vi "Read Dashboard Variables.vi"() -> ()   [LabVIEW 2020]
uses:
  <vilib>/Rock Robotics/Network Tables/NT Read Number.vi
  Framework/Robot Global Data.vi
  <vilib>/Rock Robotics/Network Tables/NT Read String.vi
panel:
  out "MaxDrive":dbl(slide)=0.6824817518248175 min=0.0 max=1.0 step=0.01 scale=0.0..1.0
  out "DriveK":dbl(slide)=0.26277372262773724 min=0.0 max=1.0 step=0.05 scale=0.0..1.0
  out "Limelight Goal Area":dbl(slide)=14.8723 min=0.1 max=25.0 step=0.25 scale=0.0..25.0
  out "AimDeadband":dbl min=0.0 max=10.0 step=0.25
  out "MinSteerCommand":dbl(slide)=0.2717391304347826 min=0.0 max=0.5 step=0.05 scale=0.0..0.5
  out "SteeringK":dbl(slide)=0.025362318840579712 min=0.0 max=0.25 step=0.01 scale=0.0..0.25
  out "Shooter Setpoint Reverse":dbl=0.8 format="%#_13g"
  out "Transfer Release Setpoint Reverse":dbl
  out "Intake Reverse Setpoint":dbl=0.8 format="%#_13g"
  out "Reverse Duration":dbl=3.0 format="%#_13g"
  out "Intake Sped Up Setpoint":dbl=0.8 format="%#_13g"
  out "Intake Sped Up Duration":dbl=3.0 format="%#_13g"
  out "Custom MaxSpeedSlow (0.6)":dbl=0.6
  out "Transfer Release Duration":dbl
  out "Transfer Up Duration":dbl
  out "Pivot Duration":dbl
  out "Pivot Right Speed":dbl
  out "Pivot Left Speed":dbl
  out "Transfer Release Setpoint":dbl
  out "Transfer Up Setpoint":dbl
  out "Intake Setpoint":dbl=0.8 format="%#_13g"
  out "Intake Duration (s)":dbl=3.0 format="%#_13g"
  out "Shooter Duration":dbl=3.0 format="%#_13g"
  out "Shooter Setpoint":dbl=0.8 format="%#_13g"
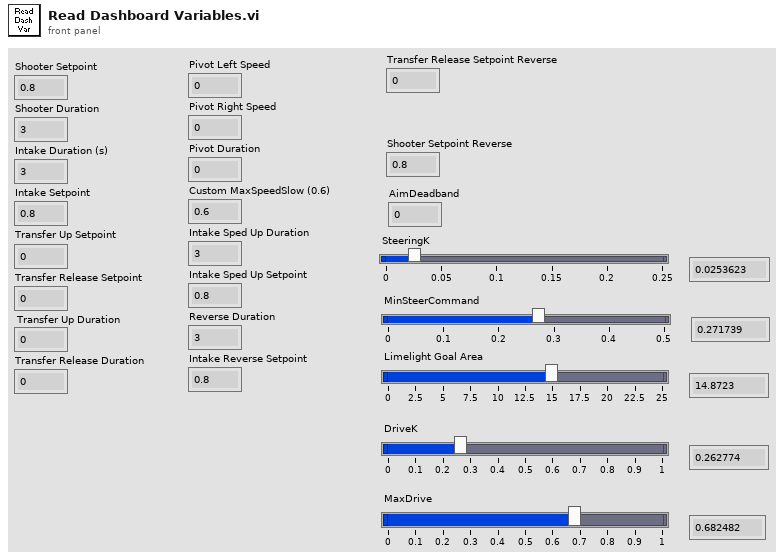
[diagram p1: front panel]
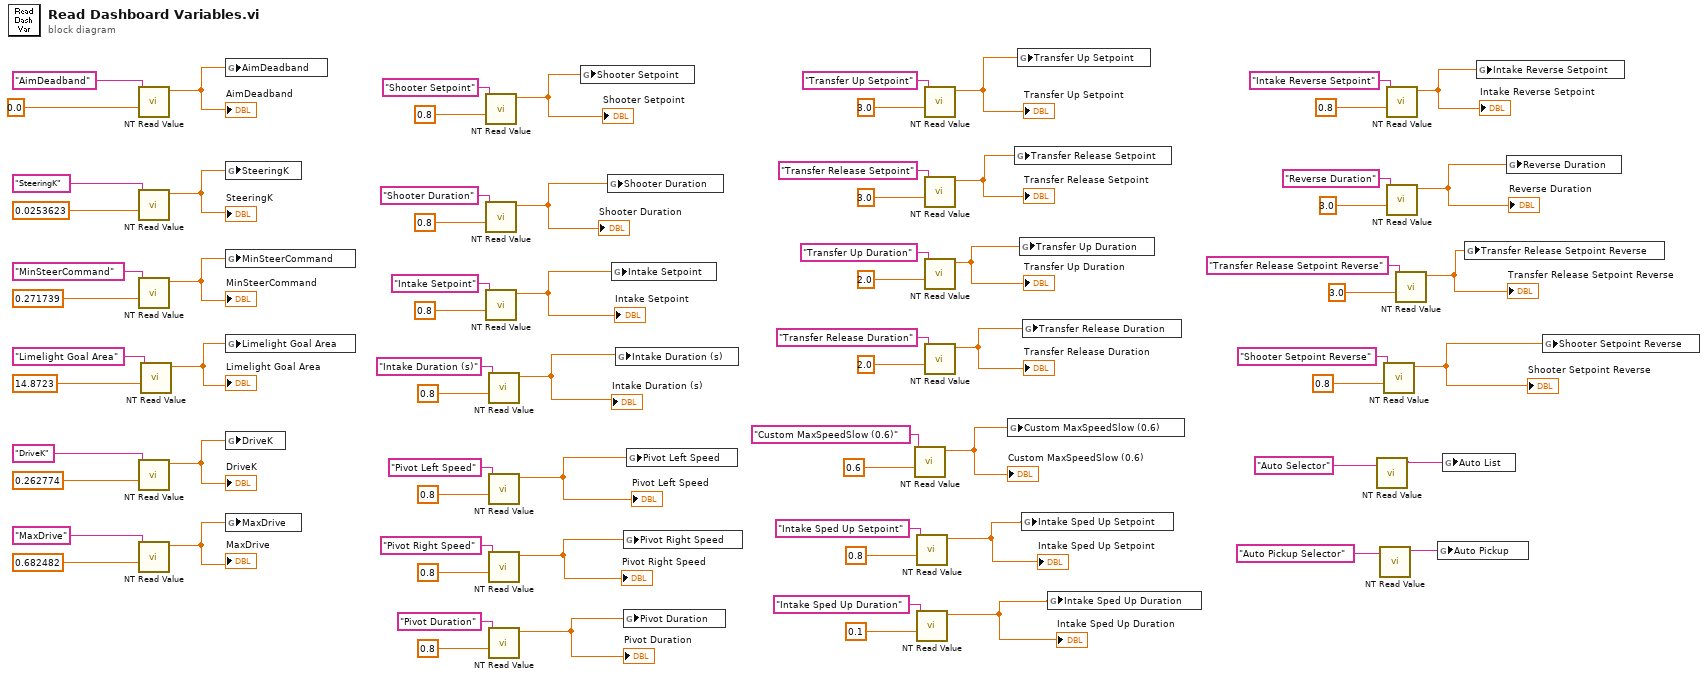
[diagram p0: block diagram]
diagram:
  n1 = call-poly <vilib>:"NT Read Value.vi"("Default Value"=0.0, "Name"="AimDeadband") -> ("Numeric"=w6:dbl)  [unwired: 8 in, 1 out]
  "AimDeadband" <- w6
  n2 = call-poly <vilib>:"NT Read Value.vi"("Default Value"=0.0253623, "Name"="SteeringK") -> ("Numeric"=w5:dbl)  [unwired: 8 in, 1 out]
  "SteeringK" <- w5
  n3 = call-poly <vilib>:"NT Read Value.vi"("Default Value"=0.271739, "Name"="MinSteerCommand") -> ("Numeric"=w4:dbl)  [unwired: 8 in, 1 out]
  "MinSteerCommand" <- w4
  n4 = call-poly <vilib>:"NT Read Value.vi"("Default Value"=0.262774, "Name"="DriveK") -> ("Numeric"=w2:dbl)  [unwired: 8 in, 1 out]
  "DriveK" <- w2
  n5 = call-poly <vilib>:"NT Read Value.vi"("Default Value"=0.682482, "Name"="MaxDrive") -> ("Numeric"=w1:dbl)  [unwired: 8 in, 1 out]
  "MaxDrive" <- w1
  n6 = call-poly <vilib>:"NT Read Value.vi"("Default Value"=14.8723, "Name"="Limelight Goal Area") -> ("Numeric"=w3:dbl)  [unwired: 8 in, 1 out]
  "Limelight Goal Area" <- w3
  n7 = global write "Robot Global Data.vi" "AimDeadband"(w6) -> ()
  n8 = global write "Robot Global Data.vi" "SteeringK"(w5) -> ()
  n9 = global write "Robot Global Data.vi" "MinSteerCommand"(w4) -> ()
  n10 = global write "Robot Global Data.vi" "Limelight Goal Area"(w3) -> ()
  n11 = global write "Robot Global Data.vi" "DriveK"(w2) -> ()
  n12 = global write "Robot Global Data.vi" "MaxDrive"(w1) -> ()
  n13 = call-poly <vilib>:"NT Read Value.vi"("Default Value"=0.8, "Name"="Shooter Setpoint") -> ("Numeric"=w74:dbl)  [unwired: 8 in, 1 out]
  "Shooter Setpoint" <- w74
  n14 = call-poly <vilib>:"NT Read Value.vi"("Default Value"=0.8, "Name"="Shooter Duration") -> ("Numeric"=w71:dbl)  [unwired: 8 in, 1 out]
  "Shooter Duration" <- w71
  n15 = call-poly <vilib>:"NT Read Value.vi"("Default Value"=0.8, "Name"="Intake Setpoint") -> ("Numeric"=w66:dbl)  [unwired: 8 in, 1 out]
  "Intake Setpoint" <- w66
  n16 = call-poly <vilib>:"NT Read Value.vi"("Default Value"=0.8, "Name"="Intake Duration (s)") -> ("Numeric"=w65:dbl)  [unwired: 8 in, 1 out]
  "Intake Duration (s)" <- w65
  n17 = call-poly <vilib>:"NT Read Value.vi"("Default Value"=0.8, "Name"="Pivot Left Speed") -> ("Numeric"=w54:dbl)  [unwired: 8 in, 1 out]
  "Pivot Left Speed" <- w54
  n18 = call-poly <vilib>:"NT Read Value.vi"("Default Value"=0.8, "Name"="Pivot Right Speed") -> ("Numeric"=w55:dbl)  [unwired: 8 in, 1 out]
  "Pivot Right Speed" <- w55
  n19 = call-poly <vilib>:"NT Read Value.vi"("Default Value"=0.8, "Name"="Pivot Duration") -> ("Numeric"=w56:dbl)  [unwired: 8 in, 1 out]
  "Pivot Duration" <- w56
  n20 = global write "Robot Global Data.vi" "Shooter Setpoint"(w74) -> ()
  n21 = global write "Robot Global Data.vi" "Shooter Duration"(w71) -> ()
  n22 = global write "Robot Global Data.vi" "Intake Setpoint"(w66) -> ()
  n23 = global write "Robot Global Data.vi" "Intake Duration (s)"(w65) -> ()
  n24 = global write "Robot Global Data.vi" "Pivot Right Speed"(w55) -> ()
  n25 = global write "Robot Global Data.vi" "Pivot Duration"(w56) -> ()
  n26 = global write "Robot Global Data.vi" "Pivot Left Speed"(w54) -> ()
  n27 = call-poly <vilib>:"NT Read Value.vi"("Default Value"=0.6, "Name"="Custom MaxSpeedSlow (0.6)") -> ("Numeric"=w37:dbl)  [unwired: 8 in, 1 out]
  "Custom MaxSpeedSlow (0.6)" <- w37
  n28 = call-poly <vilib>:"NT Read Value.vi"("Default Value"=0.8, "Name"="Intake Sped Up Setpoint") -> ("Numeric"=w32:dbl)  [unwired: 8 in, 1 out]
  "Intake Sped Up Setpoint" <- w32
  n29 = call-poly <vilib>:"NT Read Value.vi"("Default Value"=0.1, "Name"="Intake Sped Up Duration") -> ("Numeric"=w31:dbl)  [unwired: 8 in, 1 out]
  "Intake Sped Up Duration" <- w31
  n30 = call-poly <vilib>:"NT Read Value.vi"("Default Value"=3.0, "Name"="Transfer Up Setpoint") -> ("Numeric"=w47:dbl)  [unwired: 8 in, 1 out]
  "Transfer Up Setpoint" <- w47
  n31 = call-poly <vilib>:"NT Read Value.vi"("Default Value"=3.0, "Name"="Transfer Release Setpoint") -> ("Numeric"=w46:dbl)  [unwired: 8 in, 1 out]
  "Transfer Release Setpoint" <- w46
  n32 = call-poly <vilib>:"NT Read Value.vi"("Default Value"=2.0, "Name"="Transfer Up Duration") -> ("Numeric"=w44:dbl)  [unwired: 8 in, 1 out]
  "Transfer Up Duration" <- w44
  n33 = call-poly <vilib>:"NT Read Value.vi"("Default Value"=2.0, "Name"="Transfer Release Duration") -> ("Numeric"=w45:dbl)  [unwired: 8 in, 1 out]
  "Transfer Release Duration" <- w45
  n34 = global write "Robot Global Data.vi" "Custom MaxSpeedSlow (0.6)"(w37) -> ()
  n35 = global write "Robot Global Data.vi" "Transfer Release Setpoint"(w46) -> ()
  n36 = global write "Robot Global Data.vi" "Transfer Up Setpoint"(w47) -> ()
  n37 = global write "Robot Global Data.vi" "Transfer Up Duration"(w44) -> ()
  n38 = global write "Robot Global Data.vi" "Intake Sped Up Setpoint"(w32) -> ()
  n39 = global write "Robot Global Data.vi" "Transfer Release Duration"(w45) -> ()
  n40 = global write "Robot Global Data.vi" "Intake Sped Up Duration"(w31) -> ()
  n41 = call-poly <vilib>:"NT Read Value.vi"("Name"="Auto Selector") -> ("String"=w41:string)  [unwired: 9 in, 1 out]
  n42 = call-poly <vilib>:"NT Read Value.vi"("Name"="Auto Pickup Selector") -> ("String"=w40:string)  [unwired: 9 in, 1 out]
  n43 = call-poly <vilib>:"NT Read Value.vi"("Default Value"=0.8, "Name"="Shooter Setpoint Reverse") -> ("Numeric"=w19:dbl)  [unwired: 8 in, 1 out]
  "Shooter Setpoint Reverse" <- w19
  n44 = call-poly <vilib>:"NT Read Value.vi"("Default Value"=0.8, "Name"="Intake Reverse Setpoint") -> ("Numeric"=w25:dbl)  [unwired: 8 in, 1 out]
  "Intake Reverse Setpoint" <- w25
  n45 = call-poly <vilib>:"NT Read Value.vi"("Default Value"=3.0, "Name"="Reverse Duration") -> ("Numeric"=w26:dbl)  [unwired: 8 in, 1 out]
  "Reverse Duration" <- w26
  n46 = call-poly <vilib>:"NT Read Value.vi"("Default Value"=3.0, "Name"="Transfer Release Setpoint Reverse") -> ("Numeric"=w22:dbl)  [unwired: 8 in, 1 out]
  "Transfer Release Setpoint Reverse" <- w22
  n47 = global write "Robot Global Data.vi" "Auto Pickup"(w40) -> ()
  n48 = global write "Robot Global Data.vi" "Auto List"(w41) -> ()
  n49 = global write "Robot Global Data.vi" "Transfer Release Setpoint Reverse"(w22) -> ()
  n50 = global write "Robot Global Data.vi" "Intake Reverse Setpoint"(w25) -> ()
  n51 = global write "Robot Global Data.vi" "Reverse Duration"(w26) -> ()
  n52 = global write "Robot Global Data.vi" "Shooter Setpoint Reverse"(w19) -> ()
